vi "Q -- interval count - auto.vi"(6 "interval (sec)":dbl=nan, 7 "action":T1, 11 "timer ref":refnum<vi>) -> (1 "tic":bool, 2 "tic state":enum16{"knock-knock", "none"}(ring), 3 "timer out":refnum<vi>)   [LabVIEW 2010]
uses:
  countdown control.ctl
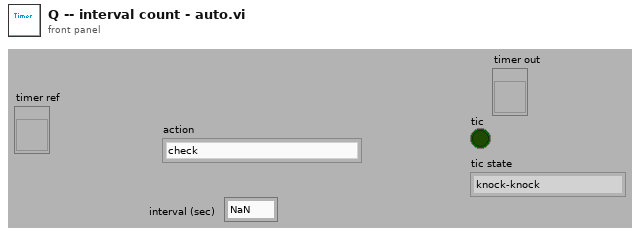
[diagram p1: front panel]
types:
  T1 = typedef "countdown control.ctl" = enum16{"check", "start", "reset"}
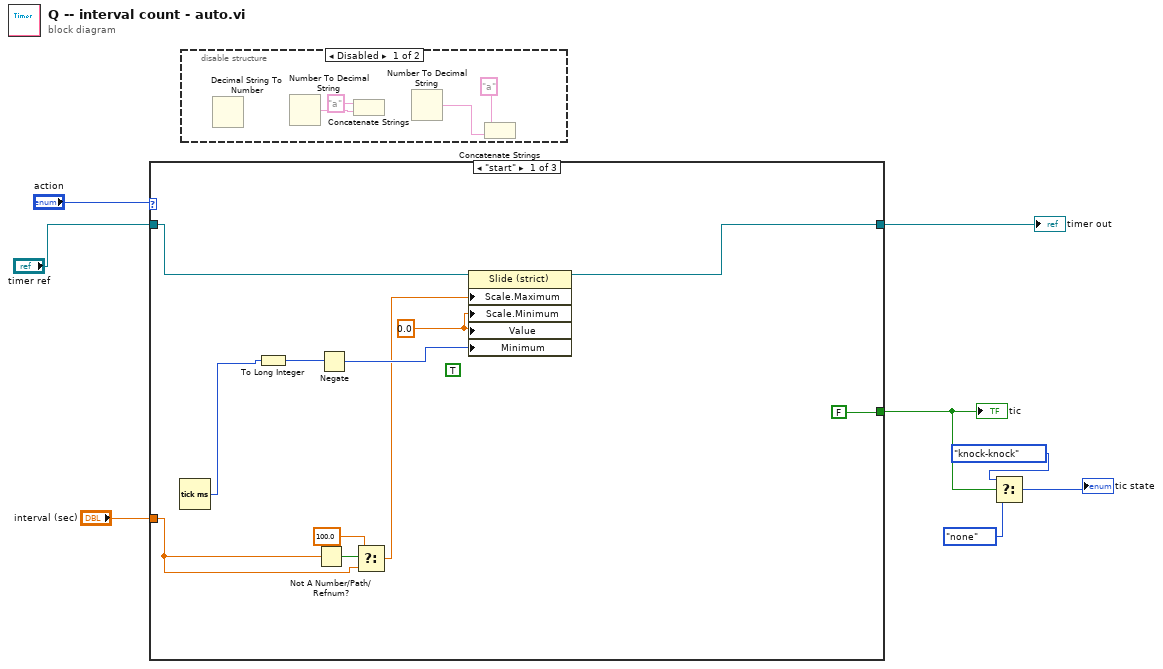
[diagram p0: block diagram]
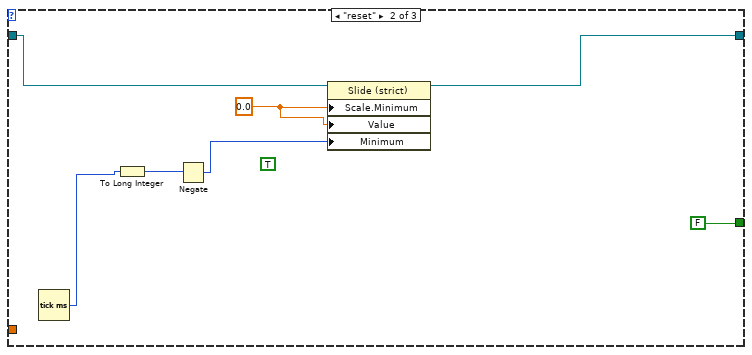
[diagram p3: hidden frame]
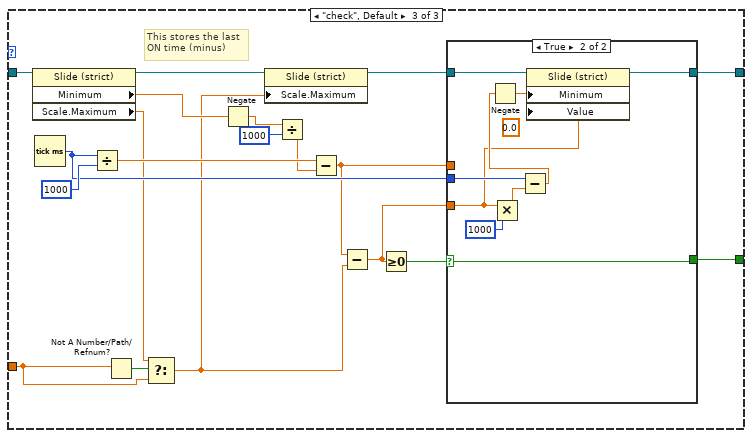
[diagram p4: hidden frame]
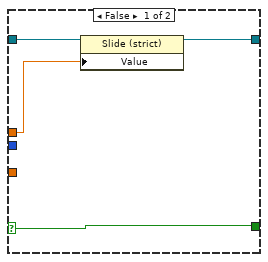
[diagram p5: hidden frame]
diagram:
  n1 = case shown="\"start\"" "action" {
    tunnel: "interval (sec)" -> [w10 _ w29]
    tunnel: [FALSE FALSE w45] -> w6
    tunnel: [w16 w23 w38] -> w2
    tunnel: "timer ref" -> [w18 w25 w42]
    frame "start" {
      (unwired) TRUE
      w17 = 0.0 ("Thermometer")
      n2 = Tick Count (ms)() -> (millisecond timer value=w14:u32)
      n3 = To Long Integer(number=w14) -> (32bit integer=w13:i32)
      n4 = Not A Number/Path/Refnum?(number/path/refnum=w10) -> (NaN/Path/Refnum?=w12:bool)
      n5 = Negate(x=w13) -> (-x=w15:i32)
      n6 = Select(t=100.0, s=w12, f=w10) -> (s? t:f=w9:dbl)
      n7 = property class="Slide (strict)"(reference=w18, "Scale.Maximum"=w9, "Scale.Minimum"=w17, "Value"=w17, "Minimum"=w15) -> (reference out=w16:refnum<vi>)  [unwired: 1 in, 1 out]
    }
    frame "reset" {
      (unwired) TRUE
      w24 = 0.0 ("Thermometer")
      n8 = Tick Count (ms)() -> (millisecond timer value=w21:u32)
      n9 = To Long Integer(number=w21) -> (32bit integer=w20:i32)
      n10 = Negate(x=w20) -> (-x=w22:i32)
      n11 = property class="Slide (strict)"(reference=w25, "Scale.Minimum"=w24, "Value"=w24, "Minimum"=w22) -> (reference out=w23:refnum<vi>)  [unwired: 1 in, 1 out]
    }
    frame "check", Default {
      # "This stores the last \nON time (minus)"
      n12 = property class="Slide (strict)"(reference=w42) -> (reference out=w31:refnum<vi>, "Minimum"=w34:dbl, "Scale.Maximum"=w28:dbl)  [unwired: 1 in, 1 out]
      n13 = Tick Count (ms)() -> (millisecond timer value=w39:u32)
      n14 = Divide(x=w39, y=1000) -> (x/y=w43:dbl)
      n15 = Not A Number/Path/Refnum?(number/path/refnum=w29) -> (NaN/Path/Refnum?=w32:bool)
      n16 = Select(t=w28, s=w32, f=w29) -> (s? t:f=w27:dbl)
      n17 = Negate(x=w34) -> (-x=w33:dbl)
      n18 = property class="Slide (strict)"(reference=w31, "Scale.Maximum"=w27) -> (reference out=w30:refnum<vi>)  [unwired: 1 in, 1 out]
      n19 = Divide(x=w33, y=1000) -> (x/y=w40:dbl)
      n20 = Subtract(x=w43, y=w40) -> (x-y=w37:dbl)
      n21 = Subtract(x=w37, y=w27) -> (x-y=w35:dbl)
      n22 = Greater Or Equal To 0?(x=w35) -> (x >= 0?=w36:bool)
      n23 = case shown="True" w36 {
        selector: w36 -> [w49 w58]
        tunnel: [w49 w58] -> w45
        tunnel: w37 -> [w48 _]
        tunnel: w30 -> [w46 w57]
        tunnel: w39 -> [_ w53]
        tunnel: [w47 w56] -> w38
        tunnel: w35 -> [_ w50]
        frame False {
          n24 = property class="Slide (strict)"(reference=w46, "Value"=w48) -> (reference out=w47:refnum<vi>)  [unwired: 1 in, 1 out]
        }
        frame True {
          (unwired) 0.0 ("Value")
          n25 = Multiply(x=w50, y=1000) -> (x*y=w54:dbl)
          n26 = Subtract(x=w53, y=w54) -> (x-y=w51:dbl)
          n27 = Negate(x=w51) -> (-x=w52:dbl)
          n28 = property class="Slide (strict)"(reference=w57, "Minimum"=w52, "Value"=w50) -> (reference out=w56:refnum<vi>)  [unwired: 1 in, 1 out]
        }
      }
    }
  }
  "tic" <- w6
  "timer out" <- w2
  n29 = disable-structure shown="Disabled" {
    frame Disabled {
      n30 = Decimal String To Number() -> ()  [unwired: 3 in, 2 out]
      n31 = Number To Decimal String() -> (decimal integer string=w61:string)  [unwired: 2 in]
      n32 = Concatenate Strings("a" ("string"), w61) -> ()  [unwired: 1 out]
      n33 = Number To Decimal String() -> (decimal integer string=w59:string)  [unwired: 2 in]
      n34 = Concatenate Strings("a" ("string"), w59) -> ()  [unwired: 1 out]
    }
    frame Enabled {
    }
  }
  n35 = Select(t=enum16{"knock-knock", "none"}."knock-knock" ("state"), s=w6, f=enum16{"knock-knock", "none"}."none" ("state")) -> (s? t:f=→"tic state":enum16{"knock-knock", "none"})
